vi "Request_Gserver_Update.vi"(8 "error in (no error)":errorcluster, 11 "Gviewer in":refnum<class "Gviewer.lvclass">) -> (0 "error out":errorcluster, 3 "Gviewer out":refnum<class "Gviewer.lvclass">)   [LabVIEW 2020, in "Sgraph_lib_V1.lvlib" / "Gviewer.lvclass"]
doc: "Andre Koelewijn, 16 jan 2021\n\nRequest update from Gserver.\nIf the update is a live data request, then updates will continuously be sent by Gserver.\nIf the 'Live' control is set to 'Freeze' then only update from Gserver will follow this command."
uses:
  Gviewer.lvclass
  controls/Typedef_datarequest.ctl
  controls/Typedef_Live.ctl
  Gserver/controls/Typedef_QueryType.ctl
  Gviewer.lvclass/Gviewer.ctl
  Gserver/Gserver.lvclass
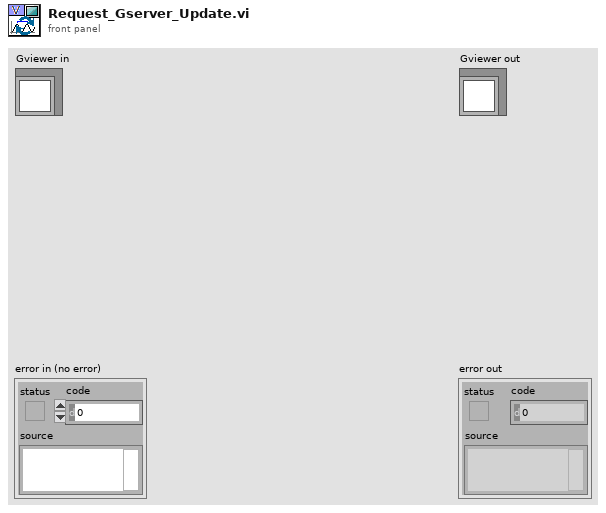
[diagram p1: front panel]
types:
  T1 = typedef "Sgraph_lib_V1.lvlib/Gserver.lvclass/Typedef_QueryType.ctl" = enum16{"Subscribe", "DataRequest", "RequestAllTags", "RequestIniPath", "FAMMstarted", "SetClientOptions", "GviewerUpdate", "OpenNewGraph", "CloseClient", "CloseAllClients", "Close Gserver", "OpenMemoryMap", "MeMapDataRequest", "MeMapDataResponse", "OpenDBeditor", "CheckDBeditorRunning", "StoppedDBeditor", "SaveDB_TAGpropRecord", "ConfirmDB_TAGpropSave"}
  T2 = typedef "Sgraph_lib_V1.lvlib/Gviewer.lvclass/Typedef_datarequest.ctl" = cluster{"Tags":string[], "Live":T3, "Time-Start":timestamp, "Time-End":timestamp, "TimeSpan":dbl, "DisplayResolution":i32}
  T3 = typedef "Sgraph_lib_V1.lvlib/Gviewer.lvclass/Typedef_Live.ctl" = enum16{"Live View", "Freeze"}
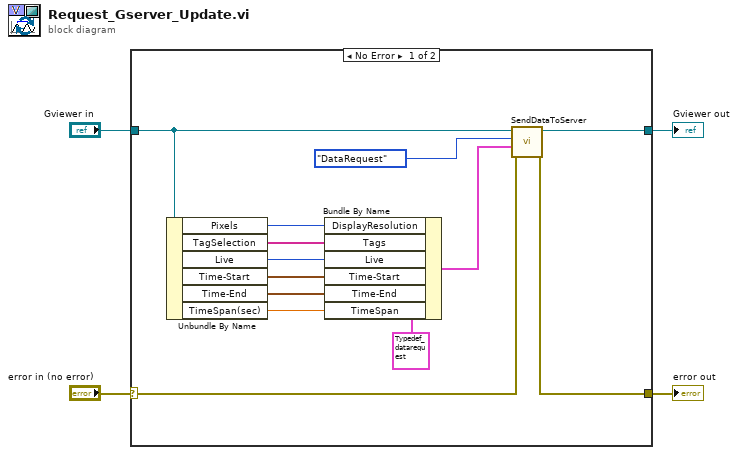
[diagram p0: block diagram]
diagram:
  n1 = case shown="No Error" "error in (no error)" {
    selector: "error in (no error)" -> [w7 w19]
    tunnel: [w6 w19] -> w3
    tunnel: [w11 w18] -> w1
    tunnel: "Gviewer in" -> [w10 w18]
    frame No Error {
      n2 = Unbundle By Name(w10) -> ("Pixels"=w5:i32, "TagSelection"=w16:string[], "Live"=w15:T3, "Time-Start"=w14:timestamp, "Time-End"=w13:timestamp, "TimeSpan(sec)"=w12:dbl)
      n3 = Bundle By Name(cluster=T2 {"Tags"=[], "Live"=enum."Live View", "Time-Start"=timestamp(0 s since 1904-01-01), "Time-End"=timestamp(0 s since 1904-01-01), "TimeSpan"=0.0, "DisplayResolution"=0} ("Cluster"), "DisplayResolution"=w5, "Tags"=w16, "Live"=w15, "Time-Start"=w14, "Time-End"=w13, "TimeSpan"=w12) -> (w8:T2)
      n4 = call "SendDataToServer.vi"("error in (no error)"=w7, "data"=w8, "Query_type"=Typedef_QueryType."DataRequest", "Gviewer in"=w10) -> ("error out"=w6:errorcluster, "Gviewer out"=w11:refnum<class "Gviewer.lvclass">)  [unwired: 6 in]
    }
    frame Error {
    }
  }
  "error out" <- w3
  "Gviewer out" <- w1
